vi "Boolean.vi"(8 "Error In":errorcluster) -> (0 "Error Out":errorcluster)   [LabVIEW 2018, in "Tests.lvlib" / "From Msgpack.lvlib"]
uses:
  From Msgpack.lvlib
  <vilib>/addons/_JKI Toolkits/Caraya/classes/Test/Test.lvclass
  src/Toolkit/Toolkit.lvlib
  <vilib>/addons/_JKI Toolkits/Caraya/classes/Assert/Assert.lvclass
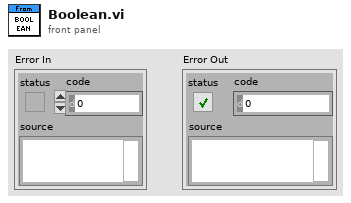
[diagram p1: front panel]
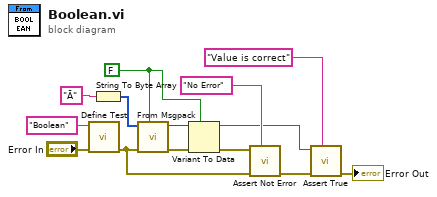
[diagram p0: block diagram]
diagram:
  w2 = FALSE
  n1 = call <vilib>:"Define Test.vi"("error in (no error)"="Error In", "Label (VI Title)"="Boolean") -> ("error out"=w8:errorcluster)  [unwired: 9 in]
  n2 = String To Byte Array(string="Ã") -> (unsigned byte array=w11:u8[])
  n3 = call "From Msgpack.vi"("Types and Defaults"=w2, "Error In"=w8, "Msgpack Data"=w11) -> ("Error Out"=w12:errorcluster, "Value"=w10:variant)  [unwired: 7 in]
  n4 = Variant To Data(error in=w12, type=w2, Variant=w10) -> (data=w1:bool, error out=w9:errorcluster)
  n5 = call <vilib>:"Assert Not Error.vi"("Label"="No Error", "error in (no error)"=w8, "Not Error?"=w9) -> ("error out"=w7:errorcluster)  [unwired: 8 in]
  n6 = call <vilib>:"Assert True.vi"("Label"="Value is correct", "error in (no error)"=w7, "True?"=w1) -> ("error out"=→"Error Out":errorcluster)  [unwired: 8 in]
